vi "Read Lossless.vi"(0 "Depth (Unlimited)":i32=-1, 1 "Timeout mS (-1)":i32=-1, 2 "FlexChannel":T2, 3 "Release (F)":bool, 4 "Restart (F)":bool, 8 "Close (F)":bool) -> (6 "Timed Out?":bool, 7 "Element":T1, 9 "Closed?":bool)   [LabVIEW 2022 SP3, in "Flex.lvlib"]
doc: "Reads data losslessly from the channel just like a Queue. The <b>Depth</b> (Max Size) of the queue can be set to a specific value to be able to throttle the writer. Be aware that causing the writer to throttle will may affect the operation of parallel readers if they expect to run unimpeded.\n\nIn order to prevent leaking references, ensure that <b>Release</b> is set to true for the last call before code stops running. If <b>Closed?</b> has returned true then the loop can cleanly close down without setting <b>Release</b> for an iteration.\n\nUnlike timeouts elsewhere in LabVIEW, if the lossless reader has been released, <b>Timed Out</b> will return true. In this way, <b>Timed Out</b> can also be used to know when to ignore the element returned while the reader is released. Once released, the reader can be restarted with the <b>Restart</b> input."
uses:
  Flex.lvlib
  ))Channel.ctl
  Element.ctl
  Queue Flags.ctl
  ChannelOp.ctl
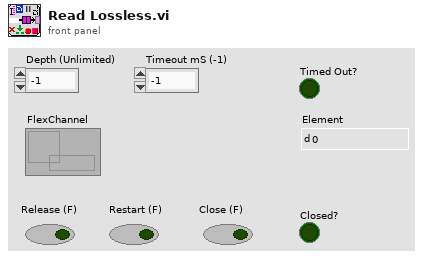
[diagram p1: front panel]
types:
  T1 = typedef "Flex.lvlib/Element.ctl" = dbl
  T2 = typedef "Flex.lvlib/))Channel.ctl" = refnum<queue>
  T3 = typedef "Flex.lvlib/Queue Flags.ctl" = u8
  T4 = typedef "Flex.lvlib/Channel Data.ctl" = cluster{"Element":refnum<data-value>, "Update":refnum<k4>, "Queue Refs":refnum<data-value>, "Event":refnum<user-event>}
  T5 = typedef "Flex.lvlib/ChannelOp.ctl" = enum16{"Get Refs", "Init", "Close", "Probe", "New Queue", "Remove Queue", "New Event"}
  T6 = typedef "Flex.lvlib/Queue Data.ctl" = cluster{"element":T1, "Flags":u8}
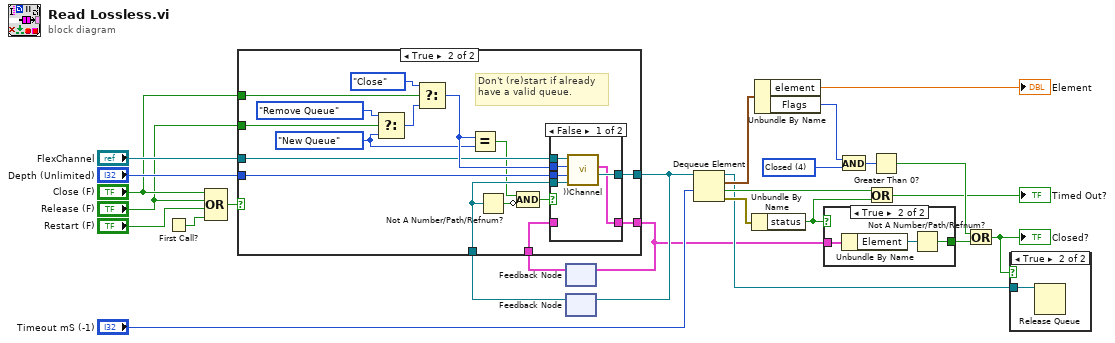
[diagram p0: block diagram]
diagram:
  w12 = T3 4 items=["Empty"=0, "Valid"=1, "Paused"=2, "Closed"=4] ("Queue Flags")
  n1 = First Call?() -> (First Call?: T/F=w18:bool)
  n2 = Compound Arithmetic op=OR("Close (F)", "Release (F)", "Restart (F)", w18) -> (w17:bool)
  n3 = feedback #1() -> (w7:T4)  [unwired: 1 in]
  n4 = feedback #2() -> (w21:refnum<queue>)  [unwired: 1 in]
  n5 = case shown="True" w17 {
    tunnel: "FlexChannel" -> [_ w42]
    tunnel: w21 -> [w27 w33]
    tunnel: "Depth (Unlimited)" -> [_ w41]
    tunnel: [w27 w40] -> w20
    tunnel: "Close (F)" -> [_ w39]
    tunnel: "Release (F)" -> [_ w38]
    tunnel: [w26 w29] -> w6
    tunnel: w7 -> [w26 w28]
    frame False {
    }
    frame True {
      w34 = ChannelOp."New Queue" ("channelOp")
      # "Don't (re)start if already have a valid queue."
      n6 = Select(t=ChannelOp."Remove Queue" ("channelOp"), s=w38, f=w34) -> (s? t:f=w36:T5)
      n7 = Select(t=ChannelOp."Close" ("channelOp"), s=w39, f=w36) -> (s? t:f=w43:T5)
      n8 = Equal?(x=w43, y=w34) -> (x = y?=w32:bool)
      n9 = Not A Number/Path/Refnum?(number/path/refnum=w33) -> (NaN/Path/Refnum?=w31:bool)
      n10 = Compound Arithmetic op=AND(w32, invert w31) -> (w30:bool)
      n11 = case shown="False" w30 {
        tunnel: w42 -> [w49 _]
        tunnel: w41 -> [w48 _]
        tunnel: [w47 w51] -> w40
        tunnel: w43 -> [w46 _]
        tunnel: w33 -> [w45 w51]
        tunnel: [w44 w50] -> w29
        tunnel: w28 -> [_ w50]
        frame False {
          n12 = call "))Channel.vi"("Remove Queue"=w45, "New Queue Depth"=w48, "channelOp"=w46, "channel in"=w49) -> ("New Queue"=w47:refnum<queue>, "Channel Data"=w44:T4)  [unwired: 3 in, 3 out]
        }
        frame True {
        }
      }
    }
  }
  n13 = feedback-in #1(w6) -> ()
  n14 = feedback-in #2(w20) -> ()
  n15 = Dequeue Element(queue=w20, timeout in ms (-1)="Timeout mS (-1)") -> (queue out=w8:refnum<queue>, element=w9:T6, timed out?=w22:bool, error out=w19:errorcluster)  [unwired: 1 in]
  n16 = Unbundle By Name(w19) -> ("status"=w1:bool)
  n17 = Unbundle By Name(w9) -> ("element"=→"Element":T1, "Flags"=w11:u8)
  n18 = case shown="True" w1 {
    tunnel: w6 -> [_ w54]
    tunnel: [_ w52] -> w5
    frame False {
    }
    frame True {
      n19 = Unbundle By Name(w54) -> ("Element"=w53:refnum<data-value>)
      n20 = Not A Number/Path/Refnum?(number/path/refnum=w53) -> (NaN/Path/Refnum?=w52:bool)
    }
  }
  n21 = And(x=w11, y=w12) -> (x .and. y?=w10:T3)
  n22 = Or(x=w22, y=w1) -> (x .or. y?=→"Timed Out?":bool)
  n23 = Greater Than 0?(x=w10) -> (x > 0?=w4:bool)
  n24 = Or(x=w4, y=w5) -> (x .or. y?=w3:bool)
  "Closed?" <- w3
  n25 = case shown="True" w3 {
    tunnel: w8 -> [_ w55]
    frame False {
    }
    frame True {
      n26 = Release Queue(queue=w55) -> ()  [unwired: 2 in, 3 out]
    }
  }
